vi "update states from tdms.vi"(8 "error in (no error)":errorcluster, 11 "5785_2_x_200MHz in":refnum<class "5785_2_x_200MHz.lvclass">) -> (0 "error out":errorcluster, 2 "tdms file mode":T1=enum."P2P - VST", 3 "5785_2_x_200MHz out":refnum<class "5785_2_x_200MHz.lvclass">)   [LabVIEW 2021]
uses:
  pulse_tx_vis/device_mode.ctl
  5785_2_x_200MHz/5785_2_x_200MHz.lvclass
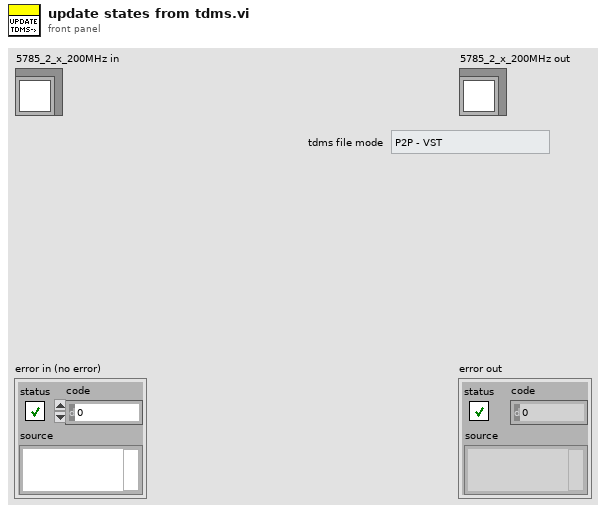
[diagram p1: front panel]
types:
  T1 = typedef "device_mode.ctl" = enum16{"USRP - 180MHz", "5785 - 2*180MHz", "5785 - 3.2GHz", "P2P - VST"}
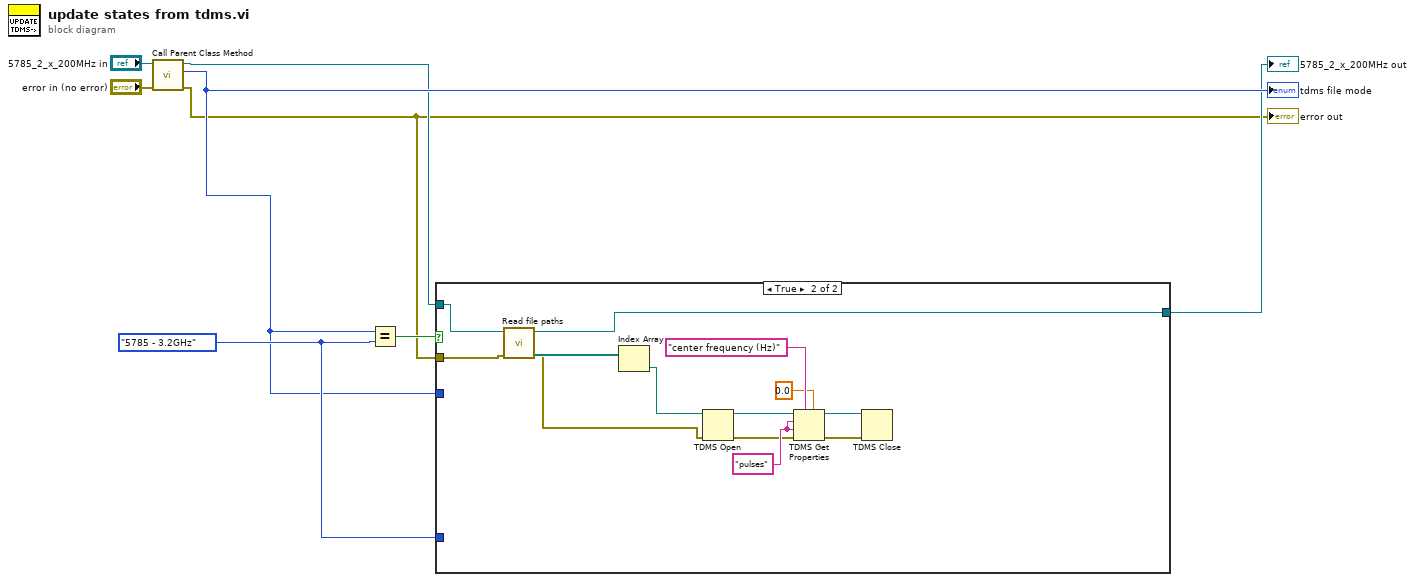
[diagram p0: block diagram]
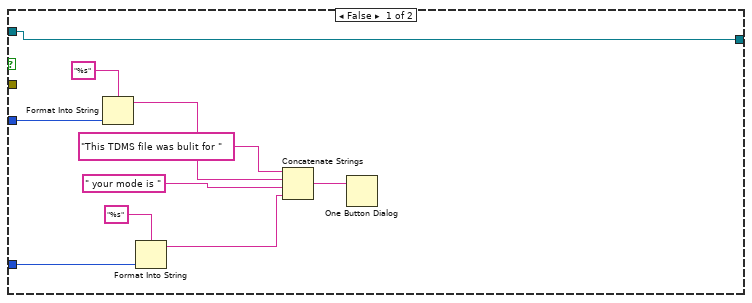
[diagram p2: hidden frame]
diagram:
  w5 = device_mode."5785 - 3.2GHz" ("Mode")
  n1 = call-parent "Call Parent Class Method"("error in (no error)"="error in (no error)", "device_type in"="5785_2_x_200MHz in") -> ("error out"=w1:errorcluster, "tdms file mode"=w4:T1, "device_type out"=w3:refnum<class "5785_2_x_200MHz.lvclass">)  [unwired: 7 in]
  "error out" <- w1
  "tdms file mode" <- w4
  n2 = Equal?(x=w4, y=w5) -> (x = y?=w6:bool)
  n3 = case shown="True" w6 {
    tunnel: w4 -> [w17 _]
    tunnel: w5 -> [w12 _]
    tunnel: w3 -> [w9 w22]
    tunnel: [w9 w19] -> w2
    tunnel: w1 -> [_ w21]
    frame False {
      n4 = Format Into String(format string="%s", w17) -> (resulting string=w16:string)  [unwired: 2 in, 1 out]
      n5 = Format Into String(format string="%s", w12) -> (resulting string=w11:string)  [unwired: 2 in, 1 out]
      n6 = Concatenate Strings("This TDMS file was bulit for " ("string"), w16, " your mode is " ("string"), w11) -> (w10:string)
      n7 = One Button Dialog(message=w10) -> ()  [unwired: 1 in, 1 out]
    }
    frame True {
      w31 = "pulses" ("channel name")
      n8 = call-dynamic "Read file paths.vi"("error in (no error)"=w21, "device_type in"=w22) -> ("error out"=w23:errorcluster, "file paths"=w25:path[], "device_type out"=w19:refnum<class "5785_2_x_200MHz.lvclass">)  [unwired: 7 in]
      n9 = Index Array(array=w25) -> (element=w24:path)  [unwired: 1 in]
      n10 = TDMS Open(8:w23, 11:w24) -> (0:w29:errorcluster, 3:w30:refnum<k34>)  [unwired: 5 in]
      n11 = TDMS Get Properties(5:0.0, 7:"center frequency (Hz)", 8:w29, 9:w31, 10:w31, 11:w30) -> (0:w26:errorcluster, 3:w27:refnum<k34>)  [unwired: 4 out]
      n12 = TDMS Close(8:w26, 11:w27) -> ()  [unwired: 2 out]
    }
  }
  "5785_2_x_200MHz out" <- w2
